vi "Add Queue.vi"(7 "Process Name":string, 8 "error in (no error)":errorcluster) -> (0 "error out":errorcluster)   [LabVIEW 2016, in "System.lvlib"]
uses:
  System.lvlib
  Controls/Control_Message Data.ctl
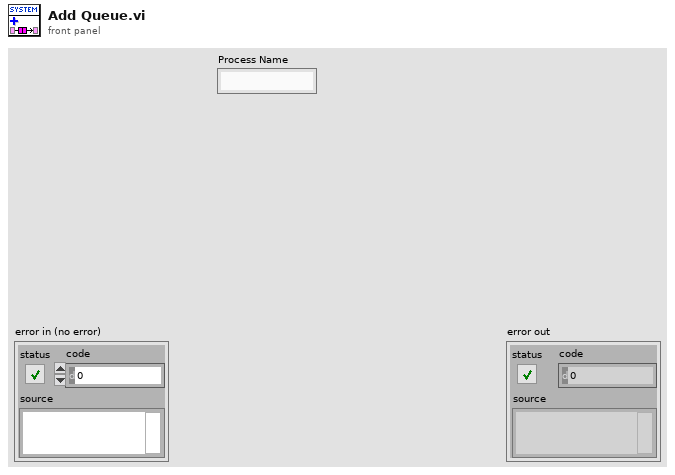
[diagram p1: front panel]
types:
  T1 = typedef "System.lvlib/Control_Message Data.ctl" = cluster{"Message":string, "Data":variant, "Sender":string}
  T2 = typedef "System.lvlib/Control_Variant Data Reference.ctl" = refnum<data-value>
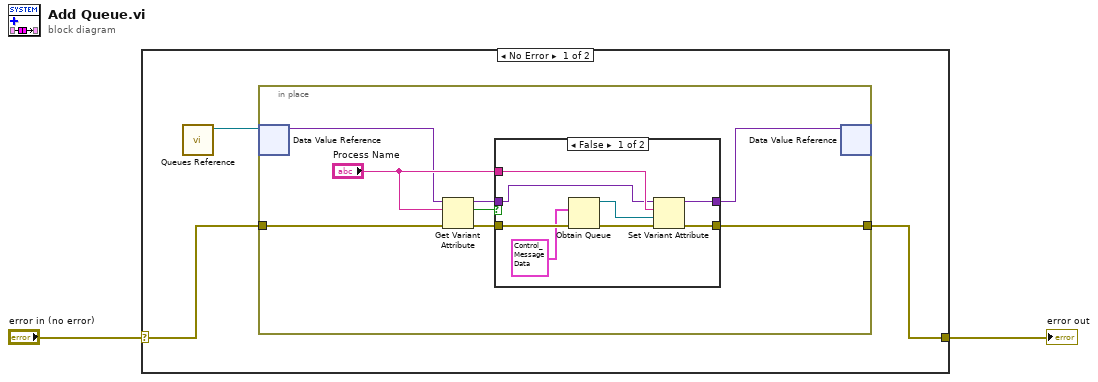
[diagram p0: block diagram]
diagram:
  n1 = case shown="No Error" "error in (no error)" {
    selector: "error in (no error)" -> [w4 w24]
    tunnel: [w3 w24] -> w1
    frame No Error {
      n2 = call "Queues Reference.vi"() -> ("Queues Reference"=w5:T2)  [unwired: 10 in, 1 out]
      n3 = in-place {
        in-place-border: w4 -> [w13]
        in-place-border: [w12] -> w3
        n4 = in-place-dvr #1(w5) -> (w7:variant)  [unwired: 1 out]
        n5 = Get Variant Attribute(Variant=w7, name="Process Name", error in=w13) -> (duplicate Variant=w10:variant, found=w11:bool, error out=w9:errorcluster)  [unwired: 1 in, 1 out]
        n6 = case shown="False" w11 {
          tunnel: w10 -> [w18 w23]
          tunnel: w9 -> [w21 w22]
          tunnel: "Process Name" -> [w19 _]
          tunnel: [w15 w23] -> w6
          tunnel: [w14 w22] -> w12
          frame False {
            n7 = Obtain Queue(element data type=T1 {"Message"="", "Data"=variant, "Sender"=""} ("Message Data"), error in (no error)=w21) -> (queue out=w16:refnum<queue>, error out=w20:errorcluster)  [unwired: 3 in, 1 out]
            n8 = Set Variant Attribute(Variant=w18, name=w19, value=w16, error in=w20) -> (Variant out=w15:variant, error out=w14:errorcluster)  [unwired: 1 out]
          }
          frame True {
          }
        }
        n9 = in-place-dvr #1(w6) -> ()  [unwired: 2 out]
      }
    }
    frame Error {
    }
  }
  "error out" <- w1
